vi "Zero.vi"(0 "VisaCluster":T1, 11 "error in (no error)":errorcluster) -> (4 "VisaCluster":T1, 8 "Answer":string, 15 "error out":errorcluster)   [LabVIEW 2014, in "FH 55.lvlib"]
doc: "The VI starts the function Zero.\n\n Durch die Funktion Zero wird die Sonde auf 'Null' gesetzt und/oder kleine Felder (z.B. das Erdfeld) unterdrückt. Normalerweise wird dafür die Sonde in die Nullfeldkammer gesteckt."
uses:
  FH 55.lvlib
  TypeDef/VisaCluster.ctl
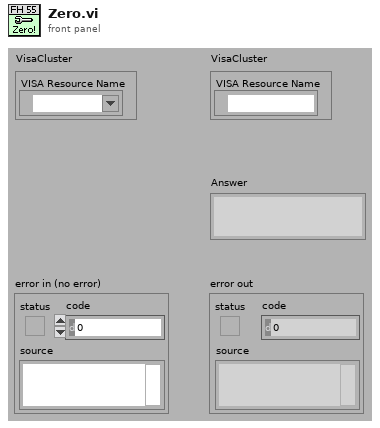
[diagram p1: front panel]
types:
  T1 = typedef "FH 55.lvlib/VisaCluster.ctl" = cluster{"VISA Resource Name":refnum<visa-resource-name>}
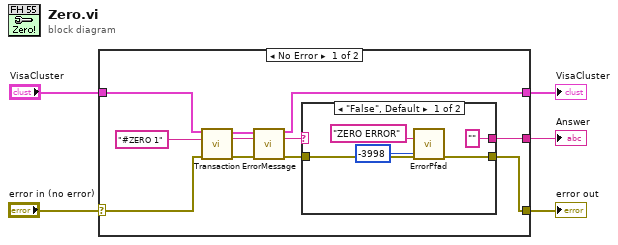
[diagram p0: block diagram]
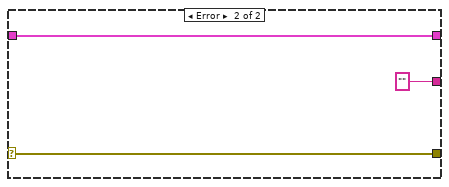
[diagram p3: hidden frame]
diagram:
  n1 = case shown="No Error" "error in (no error)" {
    selector: "error in (no error)" -> [w14 w25]
    tunnel: "VisaCluster" -> [w15 w26]
    tunnel: [w16 w26] -> w1
    tunnel: [w6 w25] -> w3
    tunnel: [w8 ""] -> w2
    frame No Error {
      n2 = call "Transaction.vi"("VisaCluster"=w15, "Command"="#ZERO 1", "error in (no error)"=w14) -> ("VisaCluster"=w11:T1, "Answer"=w12:string, "error out"=w13:errorcluster)  [unwired: 9 in, 1 out]
      n3 = call "ErrorMessage.vi"("VisaCluster"=w11, "Message In"=w12, "error in (no error)"=w13) -> ("VisaCluster"=w16:T1, "Message Out"=w9:string, "error out"=w7:errorcluster)  [unwired: 10 in]
      n4 = case shown="\"False\", Default" w9 {
        selector: w9 -> [_ w23]
        tunnel: ["" w23] -> w8
        tunnel: w7 -> [w17 w22]
        tunnel: [w20 w22] -> w6
        frame "False", Default {
          n5 = call "ErrorPfad.vi"("Message In"="ZERO ERROR", "Numeric"=-3998 ("code"), "error in (no error)"=w17) -> ("error out"=w20:errorcluster)  [unwired: 11 in, 1 out]
        }
        frame "OK\r\n" {
        }
      }
    }
    frame Error {
    }
  }
  "error out" <- w3
  "Answer" <- w2
  "VisaCluster" <- w1
